vi "AguaClara license file.vi"(1 "year":u16=2005) -> (0 "Accepted":bool)   [LabVIEW 2010]
uses:
  <vilib>/Utility/config.llb/Read Key (Boolean).vi
  <vilib>/Utility/config.llb/Write Key (Boolean).vi
  <vilib>/Utility/config.llb/NI_LVConfig.lvlib
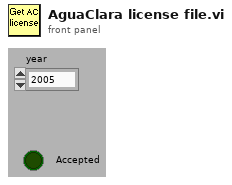
[diagram p1: front panel]
types:
  T1 = typedef "NI_LVConfig.lvlib/Config Data RefNum.ctl" = refnum<k1>
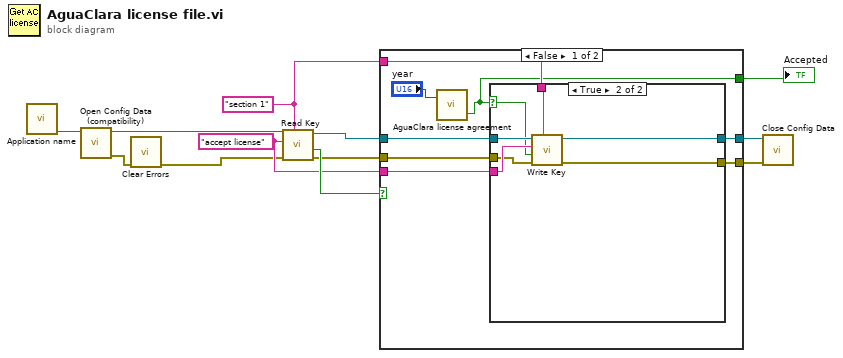
[diagram p0: block diagram]
diagram:
  w8 = "section 1" ("section")
  w9 = "accept license" ("key")
  n1 = call "Application name.vi"() -> ("Ini file path"=w3:path)  [unwired: 4 in, 3 out]
  n2 = call <vilib>:"Open Config Data (compatibility).vi"("configuration file path"=w3) -> ("error out"=w2:errorcluster, "refnum"=w12:T1)  [unwired: 8 in, 1 out]
  n3 = call <vilib>:"Clear Errors.vi"("error in (no error)"=w2) -> ("error out"=w1:errorcluster)  [unwired: 6 in]
  n4 = call-poly <vilib>:"Read Key.vi"("section"=w8, "error in (no error)"=w1, "key"=w9, "refnum"=w12) -> ("error out"=w5:errorcluster, "value"=w11:bool, "refnum out"=w10:T1)  [unwired: 4 in, 1 out]
  n5 = case shown="False" w11 {
    selector: w11 -> [_ w30]
    tunnel: w10 -> [w19 w32]
    tunnel: w9 -> [w18 _]
    tunnel: w8 -> [w17 _]
    tunnel: [w16 w32] -> w7
    tunnel: [w15 w31] -> w6
    tunnel: w5 -> [w14 w31]
    tunnel: [w13 w30] -> w4
    frame False {
      n6 = call "AguaClara license agreement.vi"("year"="year") -> ("Accepted"=w13:bool)  [unwired: 1 in, 1 out]
      n7 = case shown="True" w13 {
        selector: w13 -> [_ w27]
        tunnel: w19 -> [w22 w29]
        tunnel: w18 -> [_ w28]
        tunnel: w17 -> [_ w26]
        tunnel: [w22 w25] -> w16
        tunnel: [w21 w24] -> w15
        tunnel: w14 -> [w21 w23]
        frame False {
        }
        frame True {
          n8 = call-poly <vilib>:"Write Key.vi"("section"=w26, "error in (no error)"=w23, "value"=w27, "key"=w28, "refnum"=w29) -> ("error out"=w24:errorcluster, "refnum out"=w25:T1)  [unwired: 4 in, 1 out]
        }
      }
    }
    frame True {
    }
  }
  "Accepted" <- w4
  n9 = call <vilib>:"Close Config Data.vi"("error in (no error)"=w6, "refnum"=w7) -> ()  [unwired: 8 in, 2 out]
